vi "Get ATS Json Out.vi"(5 "extra fields in":cluster{"skipped":bool, "skip reason":string}, 6 "start timestamp in":string, 7 "test case in":string, 8 "error in":errorcluster, 9 "test time (s) in":dbl format="%#_13g", 10 "test error in":errorcluster, 11 "pass in":bool) -> (0 "error out":errorcluster, 3 "ats json out":string)   [LabVIEW 2022 SP3]
uses:
  Arcadia/Common/Framework/ATS Test Output.ctl
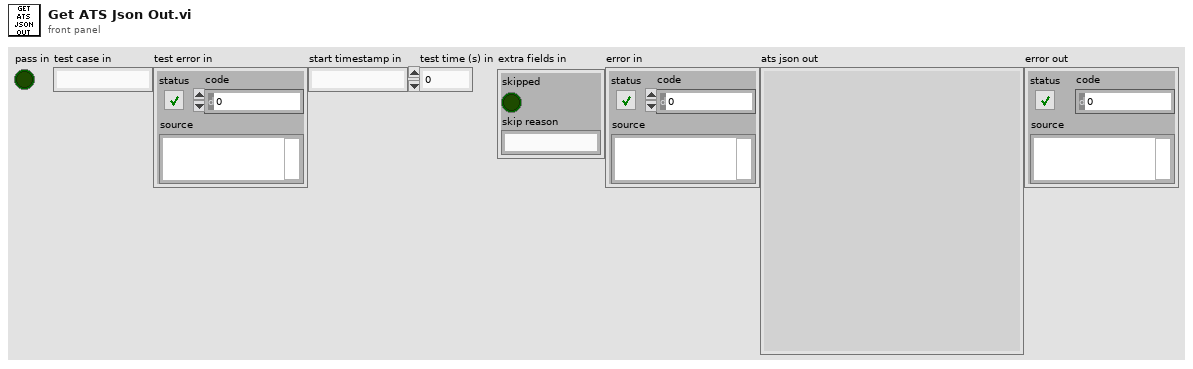
[diagram p1: front panel]
types:
  T1 = typedef "ATS Test Output.ctl" = cluster{"Test Case":string, "Pass":bool, "Skipped":bool, "Skip Reason":string, "Test Error":errorcluster, "Start Timestamp":string, "Test Time (s)":dbl, "Custom Target Name":string, "Use Custom Device List":bool, "Custom Device List":string[], "Cancel Retry":bool, "Schema Version":u32, "Schema Oldest Compatible Version":u32}
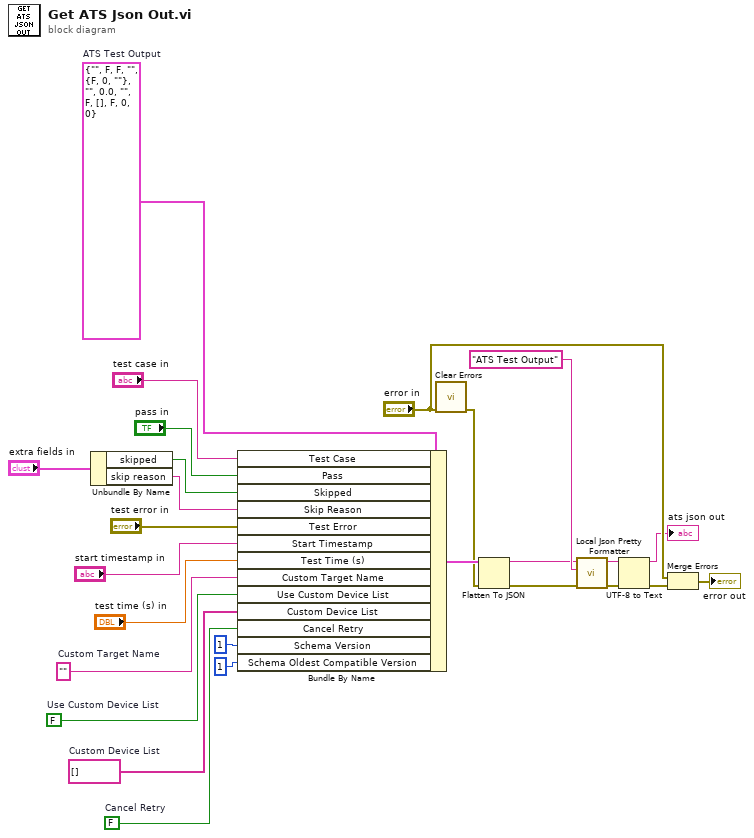
[diagram p0: block diagram]
diagram:
  w4 = ""  # Custom Target Name
  w5 = FALSE  # Cancel Retry
  w13 = string[] []  # Custom Device List
  w14 = FALSE  # Use Custom Device List
  w26 = T1 {"Test Case"="", "Pass"=FALSE, "Skipped"=FALSE, "Skip Reason"="", "Test Error"={"status"=FALSE, "code"=0, "source"=""}, "Start Timestamp"="", "Test Time (s)"=0.0, "Custom Target Name"="", "Use Custom Device List"=FALSE, "Custom Device List"=[], "Cancel Retry"=FALSE, "Schema Version"=0, "Schema Oldest Compatible Version"=0}  # ATS Test Output
  n1 = Unbundle By Name("extra fields in") -> ("skipped"=w2:bool, "skip reason"=w1:string)
  n2 = Bundle By Name(cluster=w26, "Test Case"="test case in", "Pass"="pass in", "Skipped"=w2, "Skip Reason"=w1, "Test Error"="test error in", "Start Timestamp"="start timestamp in", "Test Time (s)"="test time (s) in", "Custom Target Name"=w4, "Use Custom Device List"=w14, "Custom Device List"=w13, "Cancel Retry"=w5, "Schema Version"=u32 1, "Schema Oldest Compatible Version"=u32 1) -> (w25:T1)
  n3 = call <vilib>:"Clear Errors.vi"("error in (no error)"="error in") -> ("error out"=w23:errorcluster)  [unwired: 5 in, 1 out]
  n4 = Flatten To JSON(anything=w25, error in (no error)=w23) -> (JSON string=w19:string, 11:w24:errorcluster)  [unwired: 1 in]
  n5 = call "Local Json Pretty Formatter.vi"("error in"=w24, "data name in"="ATS Test Output" ("data name"), "json in"=w19) -> ("error out"=w9:errorcluster, "json out"=w7:string)  [unwired: 7 in]
  n6 = UTF-8 to Text(8:w9, 11:w7) -> (0:w8:errorcluster, 3:→"ats json out":string)  [unwired: 1 in]
  n7 = Merge Errors("error in", w8) -> (→"error out":errorcluster)
